vi "FTT Query Creat Cmd.vi"(3 "error in (no error)":errorcluster, 5 "DB Dispaly":T1 {"StartTime" format="%<%Y/%m/%d %H:%M>T"; "EndTime" format="%<%Y/%m/%d %H:%M>T"}) -> (0 "error out":errorcluster, 1 "Strs":string, 2 "Str":string)   [LabVIEW 2014]
uses:
  Type'def/DB Query.ctl
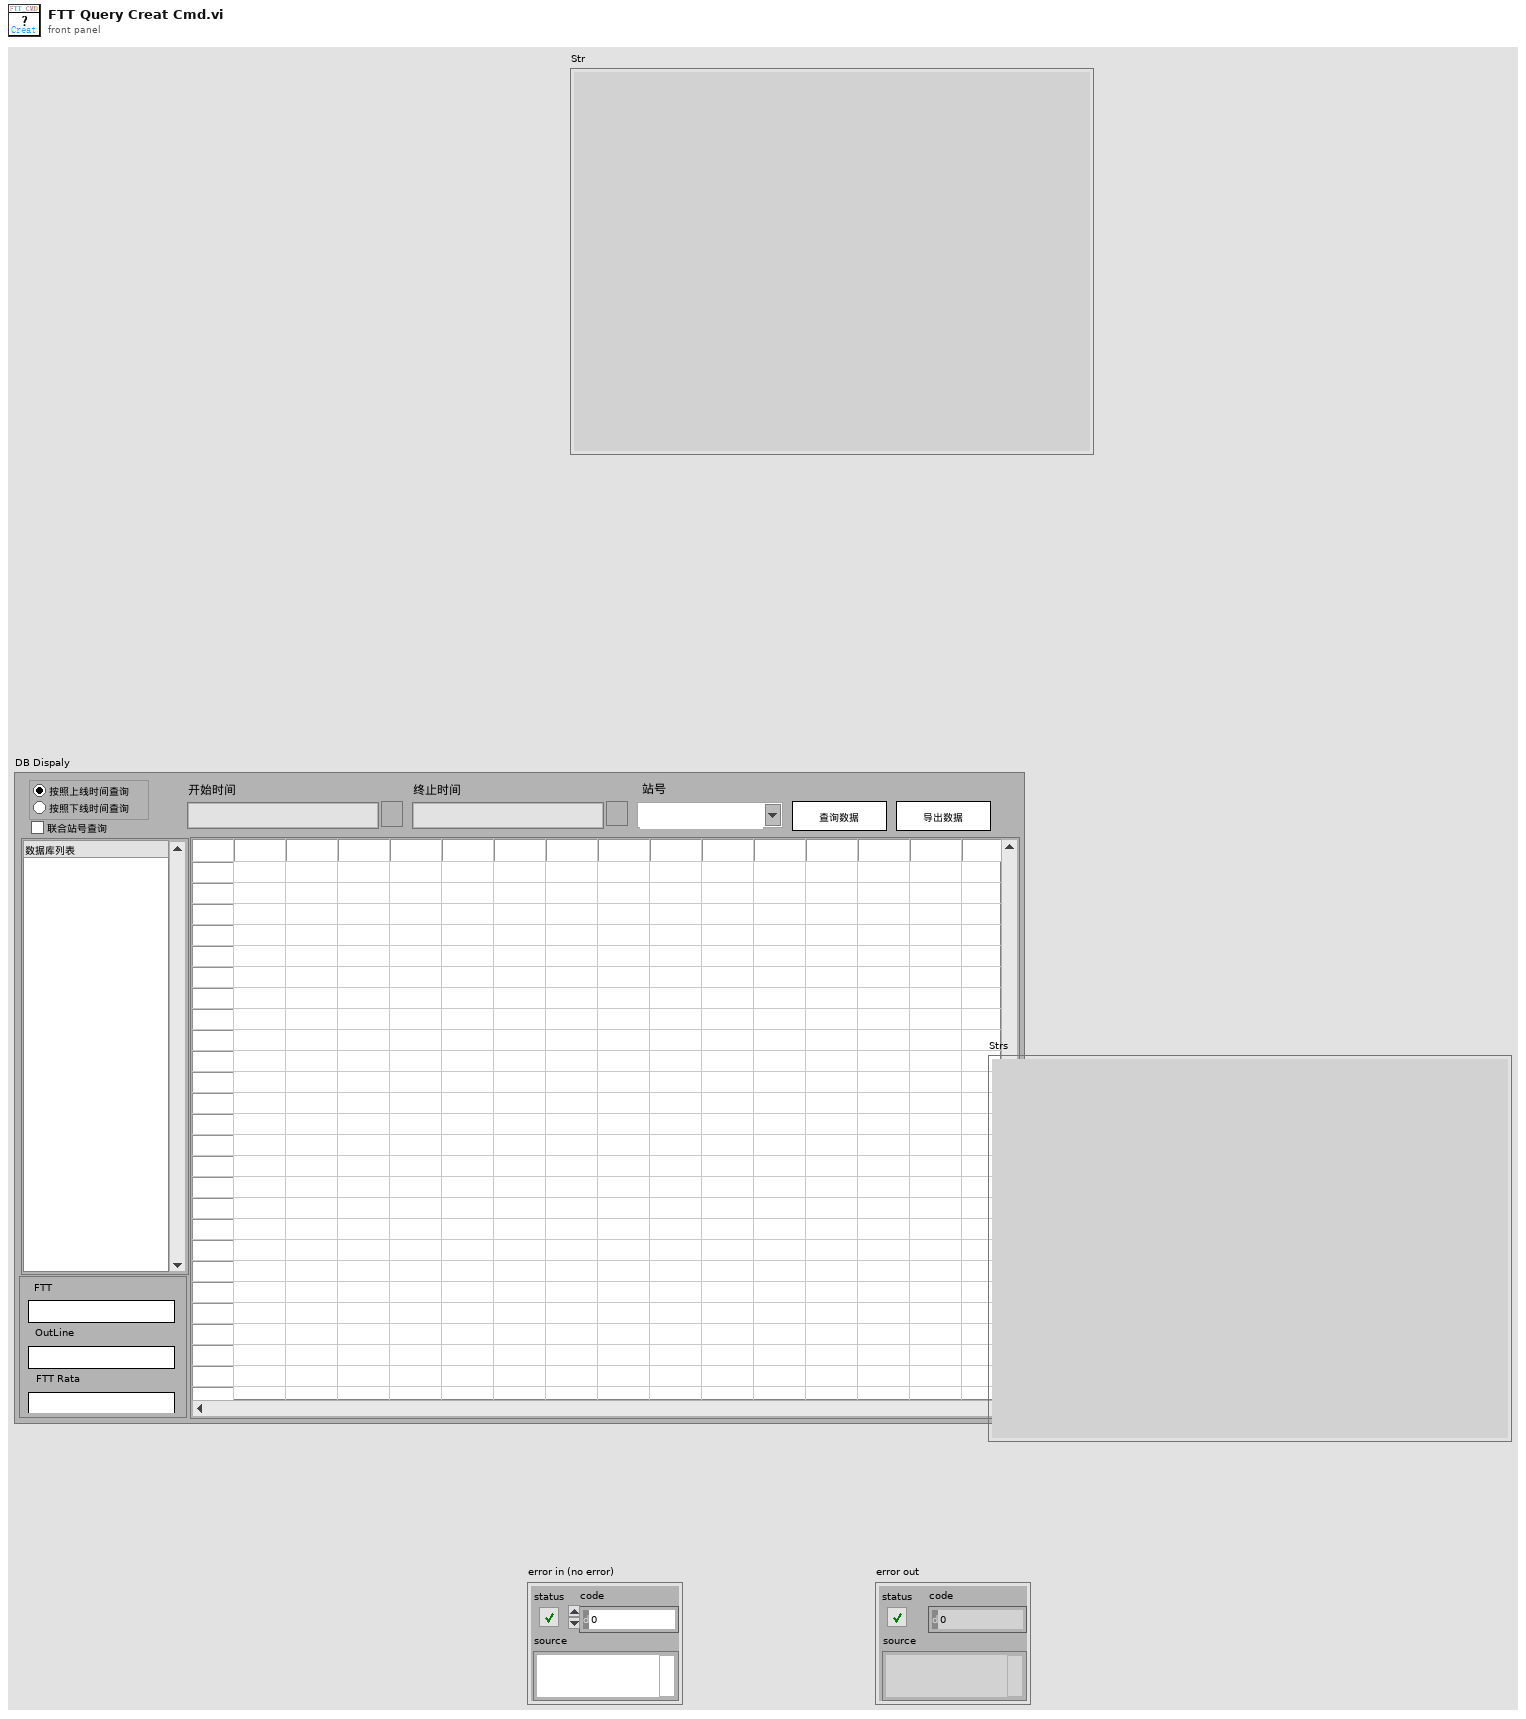
[diagram p1: front panel]
types:
  T1 = typedef "DB Query.ctl" = cluster{"Export":bool, "Query":bool, "Station.No":string, "EndTime":timestamp, "StartTime":timestamp, "FTT":cluster{"FTT":string, "OutLine":string, "FTT Rata":string}, "TableName":string, "List":string[][], "Station":bool, "QTime":enum32{"Online", "Outline"}}
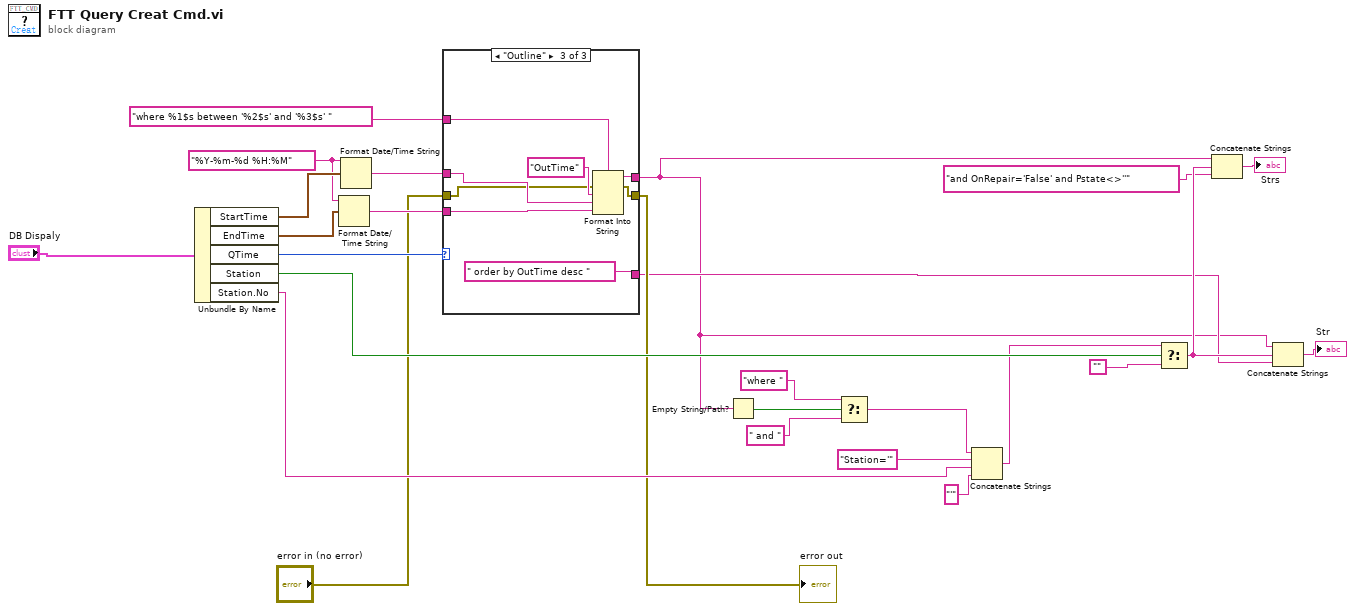
[diagram p0: block diagram]
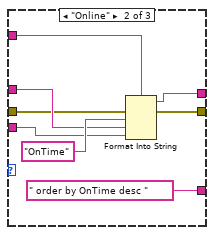
[diagram p3: hidden frame]
diagram:
  w25 = "%Y-%m-%d %H:%M" ("时间格式字符串(%c)")
  n1 = Unbundle By Name("DB Dispaly") -> ("StartTime"=w26:timestamp, "EndTime"=w24:timestamp, "QTime"=w20:enum32{"Online", "Outline"}, "Station"=w19:bool, "Station.No"=w15:string)
  n2 = Format Date/Time String(time format string (%c)=w25, seconds (now)=w24) -> (date/time string=w22:string)  [unwired: 1 in]
  n3 = Format Date/Time String(time format string (%c)=w25, seconds (now)=w26) -> (date/time string=w23:string)  [unwired: 1 in]
  n4 = case shown="\"Outline\"" w20 {
    tunnel: w23 -> [_ w33 w41]
    tunnel: w22 -> [_ w32 w40]
    tunnel: "where %1$s between '%2$s' and '%3$s' " -> [_ w35 w42]
    tunnel: [_ w31 w39] -> w1
    tunnel: [_ " order by OnTime desc " " order by OutTime desc "] -> w2
    tunnel: "error in (no error)" -> [w27 w29 w37]
    tunnel: [w27 w28 w36] -> w6
    frame Default {
    }
    frame "Online" {
      n5 = Format Into String(format string=w35, error in=w29, "OnTime" ("输入 1"), w33, w32) -> (resulting string=w31:string, error out=w28:errorcluster)  [unwired: 1 in]
    }
    frame "Outline" {
      n6 = Format Into String(format string=w42, error in=w37, "OutTime" ("输入 1"), w41, w40) -> (resulting string=w39:string, error out=w36:errorcluster)  [unwired: 1 in]
    }
  }
  "error out" <- w6
  n7 = Empty String/Path?(string/path=w1) -> (empty?=w17:bool)
  n8 = Select(t="where " ("字符串"), s=w17, f=" and ") -> (s? t:f=w11:string)
  n9 = Concatenate Strings(w11, "Station='", w15, "'" ("字符串")) -> (w10:string)
  n10 = Select(t=w10, s=w19, f="") -> (s? t:f=w4:string)
  n11 = Concatenate Strings(w1, w4, "and OnRepair='False' and Pstate<>''") -> (→"Strs":string)
  n12 = Concatenate Strings(w1, w4, w2) -> (→"Str":string)
